vi "02graba_en_panel.vi"(2 "Equipo Nº":i32, 3 "Panel":T3 {"Ultima recepción" format="%<%d/%m - %X>T"}, 4 "Paneles in":T2(array[cluster]) {"Numeric" min=1.0 max=60.0 step=1.0 format="%#2.1f"; "Ultima recepción" format="%<%d/%m - %X>T"; "Med\nPpal" format="%_4g"}) -> (1 "Paneles out":T1(array[cluster]) {"Numeric" min=1.0 max=60.0 step=1.0 format="%#2.1f"; "Ultima recepción" format="%<%d/%m - %X>T"; "Med\nPpal" format="%_4g"})   [LabVIEW 2010]
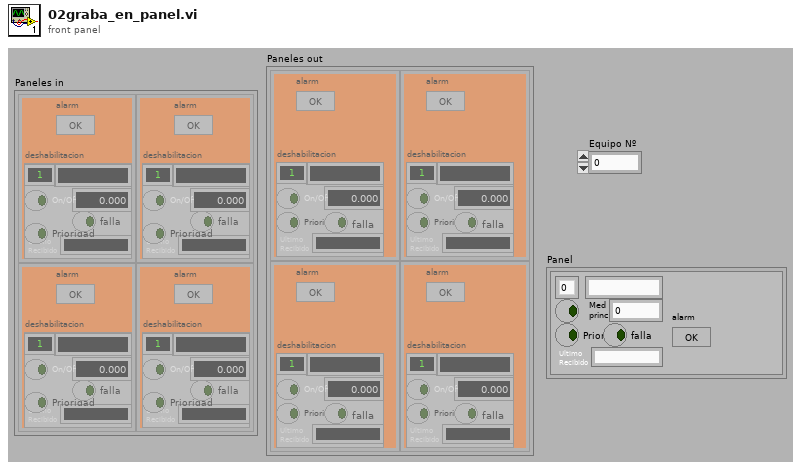
[diagram p1: front panel]
types:
  T1 = cluster{"Nombre":string, "Med\nPpal":dbl, "On/Off":bool, "Ultima recepción":timestamp, "Numeric":dbl, "deshabilitacion":bool, "Prioridad 2":bool, "falla":bool, "alarm":bool}[][]
  T2 = cluster{"Nombre":string, "Med\nPpal":dbl, "On/Off":bool, "Ultima recepción":timestamp, "Numeric":dbl, "deshabilitacion":bool, "Prioridad":bool, "falla":bool, "alarm":bool}[][]
  T3 = cluster{"Nombre":string, "Med\nprinc":dbl, "On/Off":bool, "Ultima recepción":timestamp, "Numeric":dbl, "STOP 2":bool, "Prioridad":bool, "falla":bool, "alarm":bool}
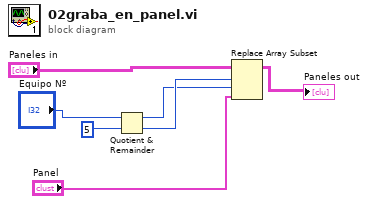
[diagram p0: block diagram]
diagram:
  n1 = Quotient & Remainder(x="Equipo Nº", y=5) -> (x-y*floor(x/y)=w1:i32, floor(x/y)=w2:i32)
  n2 = Replace Array Subset(array="Paneles in", new element="Panel", index (row)=w2, index (col)=w1) -> (→"Paneles out":T2)
